vi "loadOutcountFiles.vi"(9 "folder":string="QAMT01\\CRH3605", 11 "working directory":path=path "c:/temp") -> (1 "OK":bool, 3 "Output":string)   [LabVIEW 2012]
panel:
  out "error out":errorcluster
  in  "error in (no error)":errorcluster
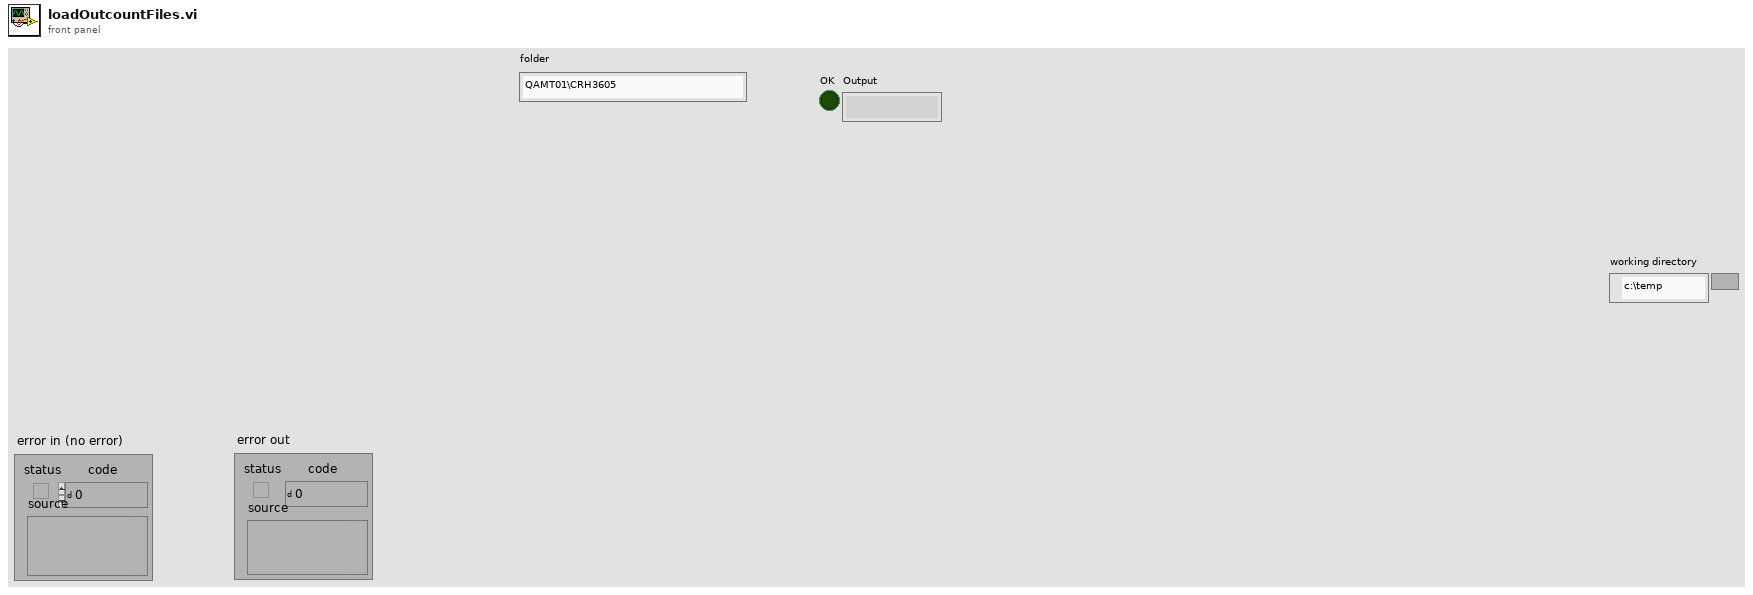
[diagram p1: front panel]
types:
  T1 = enum16{"open", "replace", "create", "open or create", "replace or create", "replace or create with confirmation"}
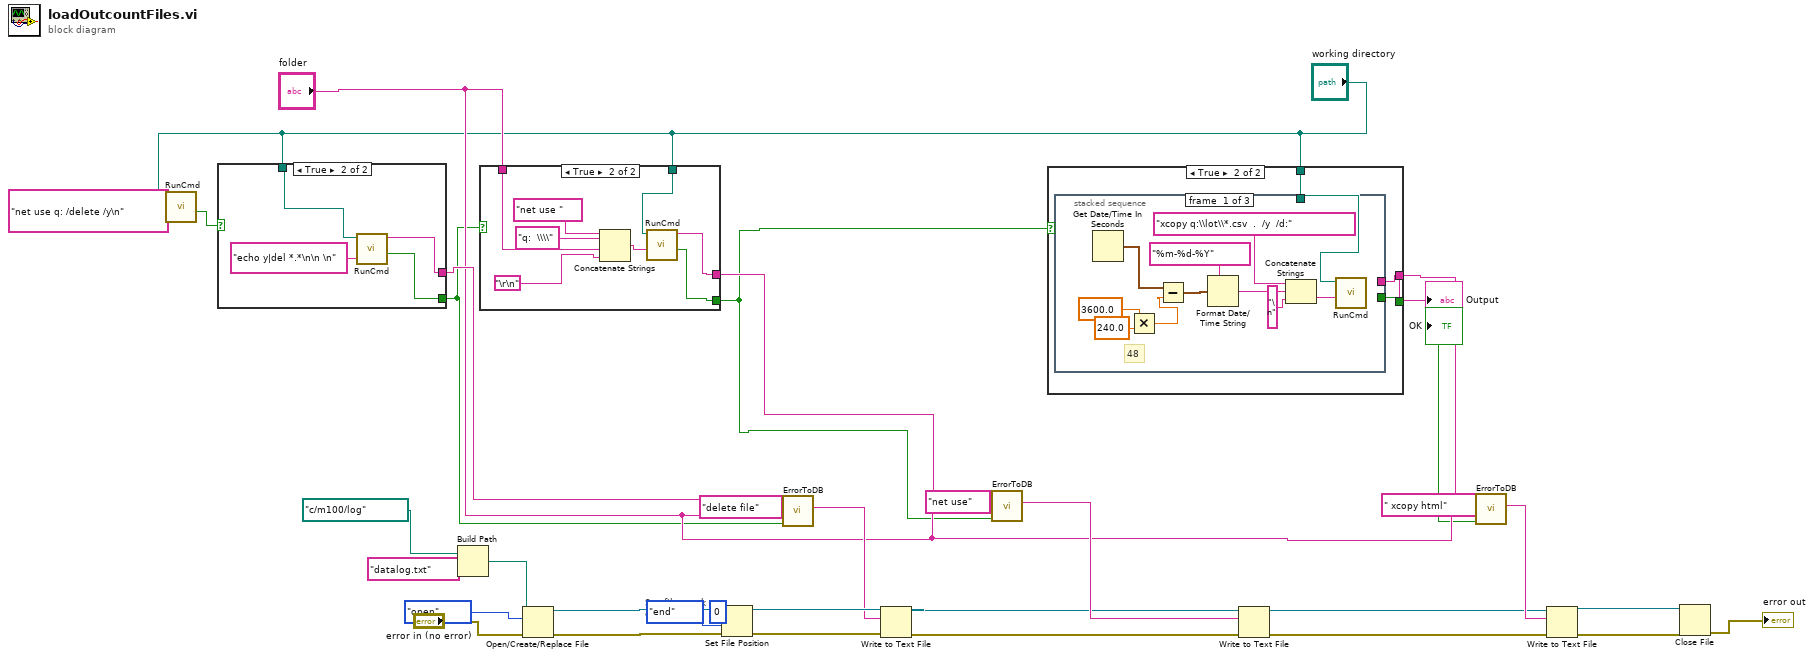
[diagram p0: block diagram]
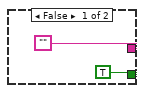
[diagram p2: hidden frame]
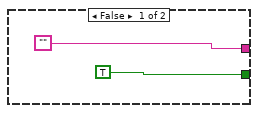
[diagram p3: hidden frame]
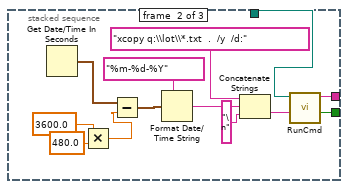
[diagram p4: hidden frame]
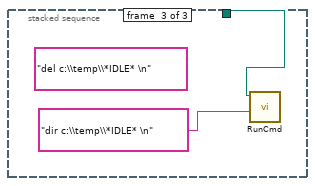
[diagram p5: hidden frame]
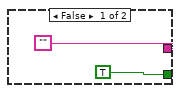
[diagram p6: hidden frame]
diagram:
  # "Set file mark to\nend of file"
  n1 = call "RunCmd.vi"("Cmd String"="net use q: /delete /y\n" ("string"), "working directory"="working directory") -> ("OK"=w20:bool)  [unwired: 8 in, 1 out]
  n2 = case shown="True" w20 {
    tunnel: [TRUE w38] -> w8
    tunnel: ["" w37] -> w15
    tunnel: "working directory" -> [_ w40]
    frame False {
    }
    frame True {
      n3 = call "RunCmd.vi"("Cmd String"="echo y|del *.*\n\n \n" ("standard input"), "working directory"=w40) -> ("OK"=w38:bool, "Output"=w37:string)  [unwired: 8 in]
    }
  }
  n4 = Build Path(base path=path "c:/m100/log", name or relative path="datalog.txt") -> (appended path=w26:path)
  n5 = case shown="True" w8 {
    tunnel: [TRUE w43] -> w1
    tunnel: ["" w44] -> w23
    tunnel: "folder" -> [_ w46]
    tunnel: "working directory" -> [_ w45]
    frame False {
    }
    frame True {
      n6 = Concatenate Strings("net use " ("string"), "q:  \\\\" ("string"), w46, "\r\n") -> (w50:string)
      n7 = call "RunCmd.vi"("Cmd String"=w50, "working directory"=w45) -> ("OK"=w43:bool, "Output"=w44:string)  [unwired: 8 in]
    }
  }
  n8 = Open/Create/Replace File(file path (use dialog)=w26, error in="error in (no error)", operation (0:open)=T1."open") -> (refnum out=w31:refnum<file>, error out=w30:errorcluster)  [unwired: 3 in, 1 out]
  n9 = Set File Position(offset (in bytes) (0)=i64 0, refnum=w31, from (0:start)=enum16{"start", "end", "current"}."end", error in=w30) -> (refnum out=w19:refnum<file>, error out=w18:errorcluster)
  n10 = call "ErrorToDB.vi"("Error"=w8, "Folder"="folder", "Command"="delete file", "Error Message"=w15) -> ("LogData"=w14:string)  [unwired: 7 in]
  n11 = Write to Text File(file (use dialog)=w19, text=w14, error in=w18) -> (refnum out=w17:refnum<file>, error out=w16:errorcluster)  [unwired: 1 in, 1 out]
  n12 = call "ErrorToDB.vi"("Error"=w1, "Folder"="folder", "Command"="net use", "Error Message"=w23) -> ("LogData"=w25:string)  [unwired: 7 in]
  n13 = case shown="True" w1 {
    tunnel: [TRUE w53] -> w9
    tunnel: ["" w54] -> w22
    tunnel: "working directory" -> [_ w55]
    frame False {
    }
    frame True {
      n14 = stacked-sequence {
        tunnel: w55 -> [w56 w69 w81]
        tunnel: [_ w68 _] -> w54
        tunnel: [_ w67 _] -> w53
        frame #0 {
          # "48"
          n15 = Get Date/Time In Seconds() -> (seconds since 1Jan1904=w57:timestamp)
          n16 = Multiply(x=3600.0, y=240.0) -> (x*y=w59:dbl)
          n17 = Subtract(x=w57, y=w59) -> (x-y=w60:timestamp)
          n18 = Format Date/Time String(time format string (%c)="%m-%d-%Y", seconds (now)=w60) -> (date/time string=w63:string)  [unwired: 1 in]
          n19 = Concatenate Strings("xcopy q:\\lot\\*.csv  .  /y  /d:" ("string"), w63, "\n" ("string")) -> (w66:string)
          n20 = call "RunCmd.vi"("Cmd String"=w66, "working directory"=w56) -> ()  [unwired: 8 in, 2 out]
        }
        frame #1 {
          n21 = Get Date/Time In Seconds() -> (seconds since 1Jan1904=w70:timestamp)
          n22 = Multiply(x=3600.0, y=480.0) -> (x*y=w72:dbl)
          n23 = Subtract(x=w70, y=w72) -> (x-y=w73:timestamp)
          n24 = Format Date/Time String(time format string (%c)="%m-%d-%Y", seconds (now)=w73) -> (date/time string=w76:string)  [unwired: 1 in]
          n25 = Concatenate Strings("xcopy q:\\lot\\*.txt  .  /y  /d:" ("string"), w76, "\n" ("string")) -> (w79:string)
          n26 = call "RunCmd.vi"("Cmd String"=w79, "working directory"=w69) -> ("OK"=w67:bool, "Output"=w68:string)  [unwired: 8 in]
        }
        frame #2 {
          (unwired) "del c:\\temp\\*IDLE* \n" ("string")
          n27 = call "RunCmd.vi"("Cmd String"="dir c:\\temp\\*IDLE* \n" ("string"), "working directory"=w81) -> ()  [unwired: 8 in, 2 out]
        }
      }
    }
  }
  "OK" <- w9
  "Output" <- w22
  n28 = Write to Text File(file (use dialog)=w17, text=w25, error in=w16) -> (refnum out=w3:refnum<file>, error out=w2:errorcluster)  [unwired: 1 in, 1 out]
  n29 = call "ErrorToDB.vi"("Error"=w9, "Folder"="folder", "Command"=" xcopy html", "Error Message"=w22) -> ("LogData"=w21:string)  [unwired: 7 in]
  n30 = Write to Text File(file (use dialog)=w3, text=w21, error in=w2) -> (refnum out=w6:refnum<file>, error out=w5:errorcluster)  [unwired: 1 in, 1 out]
  n31 = Close File(refnum=w6, error in=w5) -> (error out=→"error out":errorcluster)  [unwired: 1 out]
